vi "ReadNumbersWithCommas.vi"(8 "error in":errorcluster, 11 "file (use dialog)":path) -> (0 "error out":errorcluster, 1 "comma?":bool, 2 "text":string, 3 "fixed":string)   [LabVIEW 2022 SP3]
uses:
  Mic/Mic_Global.vi
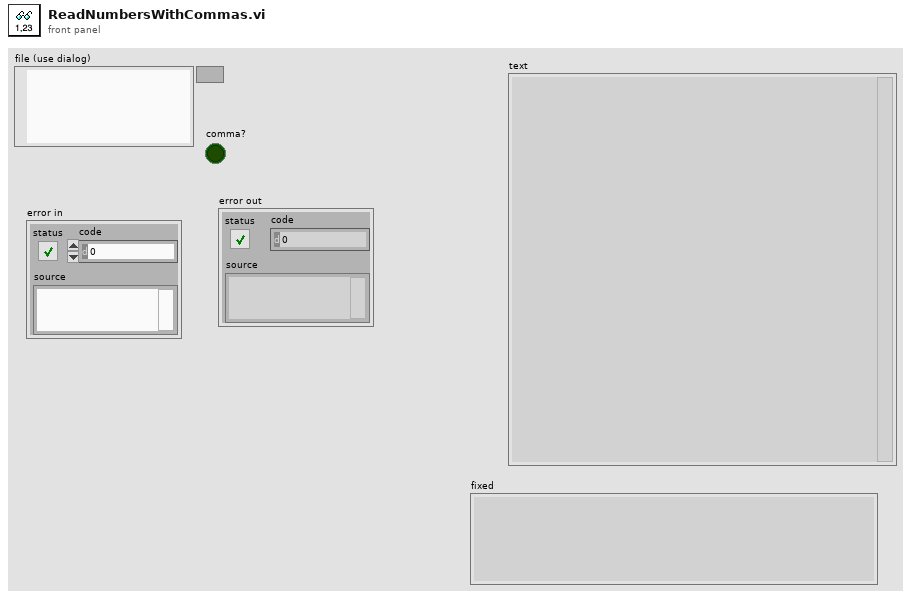
[diagram p1: front panel]
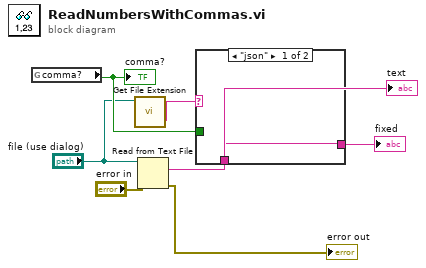
[diagram p0: block diagram]
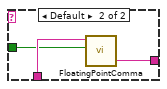
[diagram p2: hidden frame]
diagram:
  n1 = global read "Mic_Global.vi" "comma?"() -> (w4:bool)
  "comma?" <- w4
  n2 = call <vilib>:"Get File Extension.vi"("file"="file (use dialog)") -> ("unmodified file extension"=w1:string)  [unwired: 6 in, 4 out]
  n3 = Read from Text File(file (use dialog)="file (use dialog)", error in="error in") -> (text=w5:string, error out=→"error out":errorcluster)  [unwired: 2 in, 2 out]
  "text" <- w5
  n4 = case shown="\"json\"" w1 {
    tunnel: w5 -> [w8 w11]
    tunnel: w4 -> [_ w10]
    tunnel: [w8 w9] -> w3
    frame "json" {
    }
    frame Default {
      n5 = call "FloatingPointComma.vi"("Comma?"=w10, "String In"=w11) -> ("fixed"=w9:string)  [unwired: 8 in, 1 out]
    }
  }
  "fixed" <- w3
